vi "test Create New Import Aliases.vi"(8 "error in (no error)":errorcluster, 11 "TestCase in":refnum<class "Routing and Faulting Import Unit Tests.lvclass">) -> (0 "error out":errorcluster, 3 "TestCase out":refnum<class "Routing and Faulting Import Unit Tests.lvclass">)   [LabVIEW 2020, in "Routing and Faulting Import Unit Tests.lvclass"]
uses:
  Routing and Faulting Import Unit Tests.lvclass
  Shared/Alias Mapping.ctl
  Shared/Alias Endpoint.ctl
  <vilib>/addons/_JKI Toolkits/VI Tester/TestCase.llb/TestCase.lvclass
  Scripting/Routing and Faulting Scripting.lvlib
  Shared/Routing and Faulting Shared.lvlib
  C:/Program Files (x86)/National Instruments/LabVIEW 2020/vi.lib/addons/_JKI Toolkits/VI Tester/TestCase.llb/TestCase.lvclass
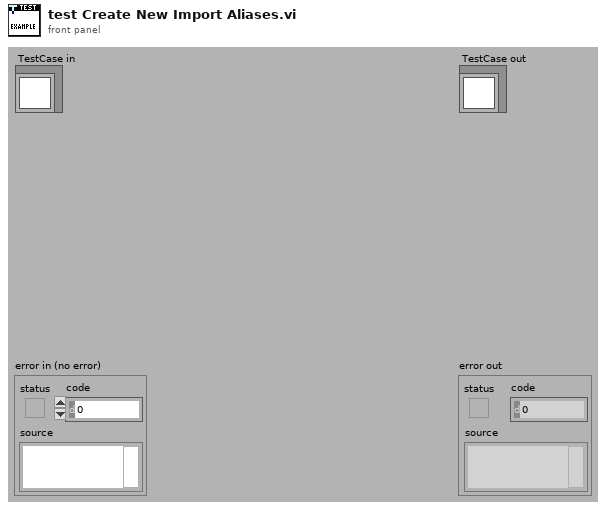
[diagram p1: front panel]
types:
  T1 = typedef "Routing and Faulting Shared.lvlib/Alias Mapping.ctl" = cluster{"Alias":string, "Endpoint":T2}
  T2 = typedef "Routing and Faulting Shared.lvlib/Alias Endpoint.ctl" = cluster{"Module Path":string, "Endpoint":string}
  T3 = typedef "Custom Device API.lvlib/Custom Device Item Ref.ctl" = u64
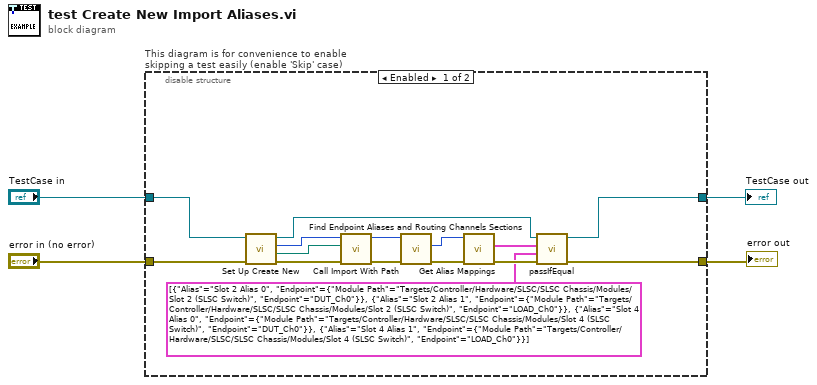
[diagram p0: block diagram]
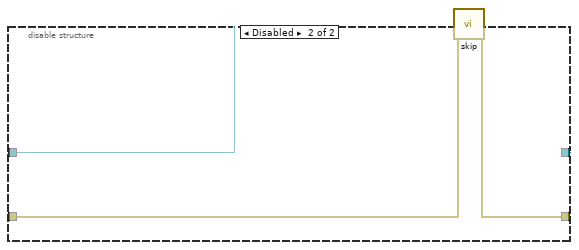
[diagram p2: hidden frame]
diagram:
  n1 = disable-structure "This diagram is for convenience to enable skipping a test easily (enable 'Skip' case)" shown="Enabled" {
    disable-tunnel: "TestCase in" -> [w13 w23]
    disable-tunnel: [w12 w21] -> w1
    disable-tunnel: [w11 w22] -> w3
    disable-tunnel: "error in (no error)" -> [w16 w20]
    frame Enabled {
      n2 = call "Set Up Create New.vi"("error in (no error)"=w16, "Test Case in"=w13) -> ("error out"=w15:errorcluster, "Import Path"=w7:path, "Routing and Faulting Custom Device Ref"=w6:T3, "Test Case out"=w10:refnum<class "Routing and Faulting Import Unit Tests.lvclass">)  [unwired: 6 in]
      n3 = call "Call Import With Path.vi"("error in (no error)"=w15, "Path"=w7, "Routing and Faulting Custom Device Ref in"=w6) -> ("error out"=w19:errorcluster, "Routing and Faulting Custom Device Ref out"=w5:T3)  [unwired: 7 in]
      n4 = call "Find Endpoint Aliases and Routing Channels Sections.vi"("error in"=w19, "routing and faulting custom device in"=w5) -> ("error out"=w18:errorcluster, "endpoint aliases"=w17:T3)  [unwired: 6 in, 2 out]
      n5 = call "Get Alias Mappings.vi"("error in"=w18, "endpoint aliases in"=w17) -> ("error out"=w14:errorcluster, "alias mappings"=w8:T1[])  [unwired: 7 in, 1 out]
      n6 = call-dynamic "passIfEqual.vi"("error in (no error)"=w14, "y"=T1[] [{"Alias"="Slot 2 Alias 0", "Endpoint"={"Module Path"="Targets/Controller/Hardware/SLSC/SLSC Chassis/Modules/Slot 2 (SLSC Switch)", "Endpoint"="DUT_Ch0"}}, {"Alias"="Slot 2 Alias 1", "Endpoint"={"Module Path"="Targets/Controller/Hardware/SLSC/SLSC Chassis/Modules/Slot 2 (SLSC Switch)", "Endpoint"="LOAD_Ch0"}}, {"Alias"="Slot 4 Alias 0", "Endpoint"={"Module Path"="Targets/Controller/Hardware/SLSC/SLSC Chassis/Modules/Slot 4 (SLSC Switch)", "Endpoint"="DUT_Ch0"}}, {"Alias"="Slot 4 Alias 1", "Endpoint"={"Module Path"="Targets/Controller/Hardware/SLSC/SLSC Chassis/Modules/Slot 4 (SLSC Switch)", "Endpoint"="LOAD_Ch0"}}] ("Alias Mappings"), "x"=w8, "TestCase in"=w10) -> ("error out"=w11:errorcluster, "TestCase out"=w12:refnum<class "Routing and Faulting Import Unit Tests.lvclass">)  [unwired: 6 in]
    }
    frame Disabled {
      # "skip test result while test is under development"
      n7 = call <vilib>:"skip.vi"("error in (no error)"=w20, "TestCase in"=w23) -> ("error out"=w22:errorcluster, "TestCase out"=w21:refnum<class "Routing and Faulting Import Unit Tests.lvclass">)  [unwired: 8 in]
    }
  }
  "error out" <- w3
  "TestCase out" <- w1
